vi "mod_QAM Transmitter Gen Symbl Map.vi"(0 "Symbol Rate, Hz":dbl=1.0 format="%.2f", 1 "Reset?":bool=TRUE, 2 "# Samples per Symbol":i32=16, 5 "M-QAM":i32=16, 7 "Message":T3={"# Guard Bits"=4, "# Sync Bits"=40, "# Message Bits"=1000, "PN sequence order"=9}, 9 "System Filter":T2={"TX Filter"=enum."Root Raised Cos", "Alpha"=0.5, "filter length"=8} {"Alpha" format="%.2f"}, 11 "error in (no error)":errorcluster, 12 "Generic Symbol Map Params":T1={"symbol values"=[[1, 17, 21, 5, 4, 20, 16, 0], [33, 49, 53, 37, 36, 52, 48, 32], [41, 57, 61, 45, 44, 60, 56, 40], [9, 25, 29, 13, 12, 28, 24, 8], [11, 27, 31, 15, 14, 30, 26, 10], [43, 59, 63, 47, 46, 62, 58, 42], [35, 51, 55, 39, 38, 54, 50, 34], [3, 19, 23, 7, 6, 22, 18, 2]], "symbol amplitudes (I)"=[-10.0, -8.0, -6.0, -4.0, 4.0, 6.0, 8.0, 10.0], "symbol amplitudes (Q)"=[10.0, 8.0, 6.0, 4.0, -4.0, -6.0, -8.0, -10.0], "gain"=108.0}, 13 "Standard/Generic":enum16{"Standard", "Generic"}(ring)) -> (4 "Output Complex Waveform":T6 {"Y" format="%.3f"; "dt" format="%^.2e"; "t0" format="%.4f"}, 6 "Signal Description":T5 {"QAM System Parameters"."symbol map" format="%.3f"; "matched filter coefficients" format="%.2f"; "pulse shaping filter coefficients" format="%.2f"; "Sync (Symbols)" format="%.2f"}, 15 "error out":errorcluster)   [LabVIEW 2020, in "niDMT.lvlib"]
doc: "This example demonstrates generation of a QAM modulated signal. You can specify characteristics of the message signal such as PN sequence order, number of guard bits, number of sync bits, and transmit filter parameters. You can extend this example to download the generated QAM signal to GPIB-based RF signal generators."
uses:
  <vilib>/addons/Modulation/niDMT.lvlib
  <vilib>/addons/Modulation/Digital/Support/Controls/QAM System Parameters.ctl
  <vilib>/addons/Modulation/Analog/controls/Complex Data Waveform.ctl
  <vilib>/addons/Modulation/Analog/support/mod_Set Error Source.vi
  <vilib>/addons/Modulation/Digital/Support/Common/Validators/mod_Generate Filter Coefficients Validate.vi
  <vilib>/addons/Modulation/Digital/General/subVIs/mod_Generate Filter Coefficients.vi
  <vilib>/addons/Modulation/Digital/General/MT Generate QAM System Parameters(M).vi
  <vilib>/addons/Modulation/niAMT.lvlib
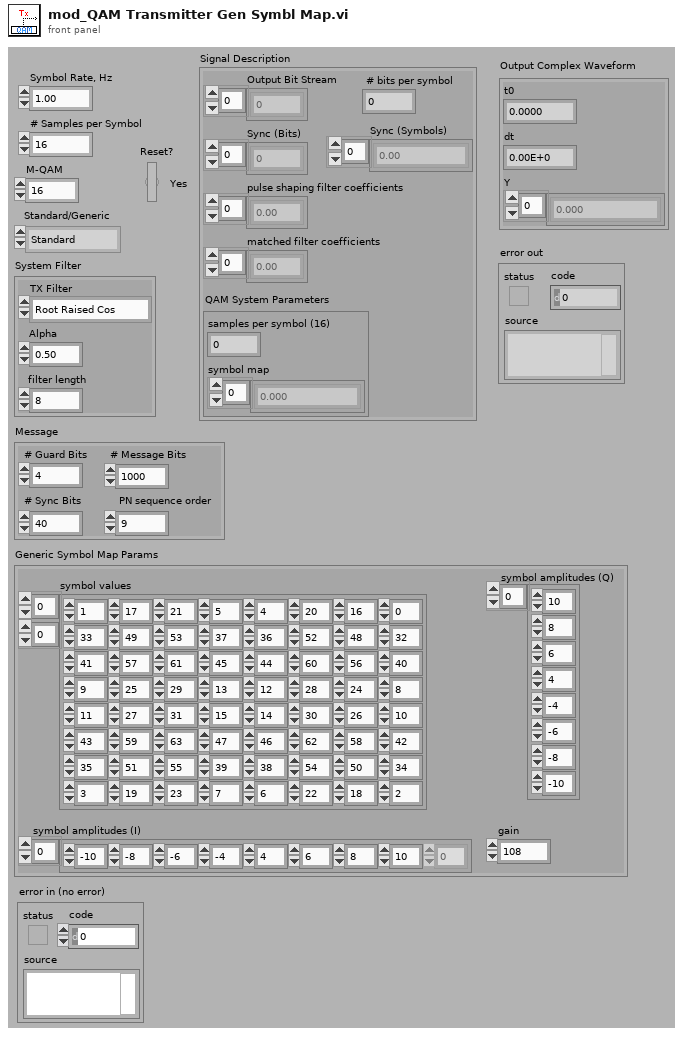
[diagram p1: front panel]
types:
  T1 = cluster{"symbol values":i32[][], "symbol amplitudes (I)":dbl[], "symbol amplitudes (Q)":dbl[], "gain":dbl}
  T2 = cluster{"TX Filter":enum16{"none", "Raised Cosine", "Root Raised Cos", "Gaussian"}, "Alpha":dbl, "filter length":i32}
  T3 = cluster{"# Guard Bits":i32, "# Sync Bits":i32, "# Message Bits":i32, "PN sequence order":i32}
  T4 = typedef "niDMT.lvlib/QAM System Parameters.ctl" = cluster{"samples per symbol (16)":i32, "symbol map":cdb[]}
  T5 = cluster{"Output Bit Stream":i8[], " # bits per symbol":i32, "Sync (Bits)":i8[], "Sync (Symbols)":cdb[], "pulse shaping filter coefficients":dbl[], "matched filter coefficients":dbl[], "QAM System Parameters":T4}
  T6 = typedef "niAMT.lvlib/Complex Data Waveform.ctl" = cluster{"t0":dbl, "dt":dbl, "Y":cdb[]}
  T7 = cluster{"Output Bit Stream":i8[], "# bits per symbol":i32, "Sync (Bits)":i8[], "Sync (Symbols)":cdb[], "pulse shaping filter coefficients":dbl[], "matched filter coefficients":dbl[], "QAM System Parameters":T4}
  T8 = enum16{"none", "Raised Cosine", "Root Raised Cos", "Gaussian"}
  T9 = cluster{"samples per symbol (16)":i32, "symbol map":cdb[]}
  T10 = cluster{"# Samples per Symbol":i32, "symbol map":cdb[]}
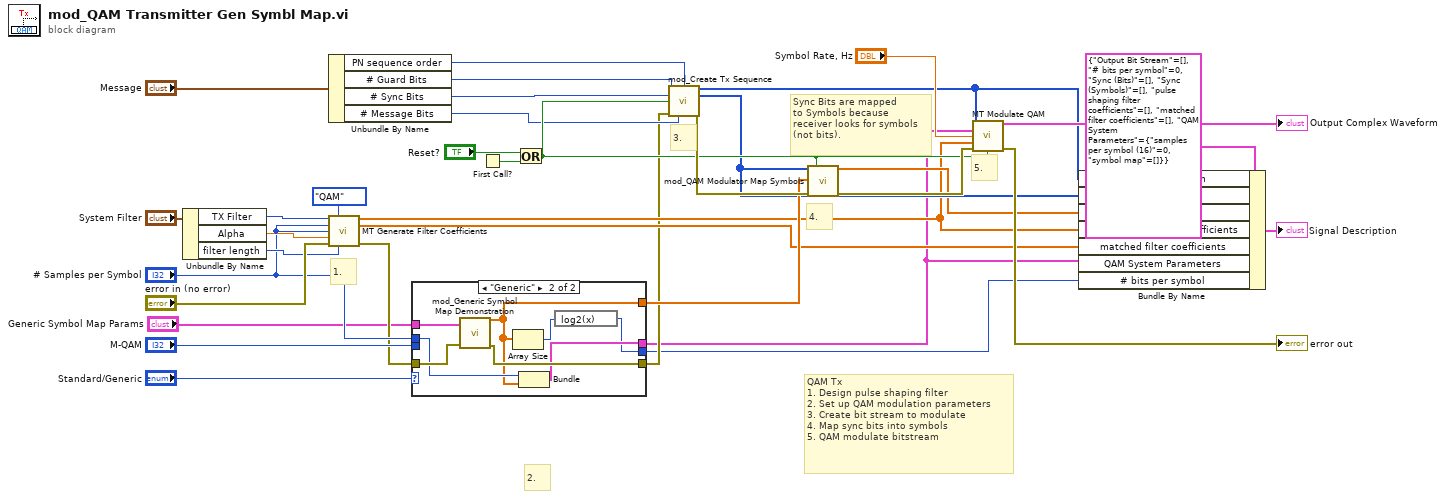
[diagram p0: block diagram]
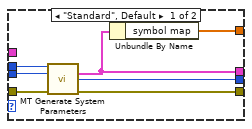
[diagram p2: hidden frame]
diagram:
  # "5."
  # "4."
  # "2."
  # "3."
  # "1."
  # "QAM Tx\n1. Design pulse shaping filter\n2. Set up QAM modulation parameters\n3. Create bit stream to modulate\n4. Map sync bits into symbols\n5. QAM modulate bitstream"
  # "Sync Bits are mapped\nto Symbols because\nreceiver looks for symbols\n(not bits)."
  n1 = Unbundle By Name("System Filter") -> ("TX Filter"=w20:T8, "Alpha"=w19:dbl, "filter length"=w18:i32)
  n2 = Unbundle By Name("Message") -> ("PN sequence order"=w12:i32, "# Guard Bits"=w24:i32, "# Sync Bits"=w23:i32, "# Message Bits"=w22:i32)
  n3 = call <vilib>:"MT Generate Filter Coefficients.vi"("pulse shaping filter (none)"=w20, "modulation type"=enum16{"FSK", "PSK", "QAM", "MSK", "PAM", "ASK"}."QAM", "pulse shaping samples per symbol (16)"="# Samples per Symbol", "matched samples per symbol (16)"="# Samples per Symbol", "filter parameter"=w19, "error in (no error)"="error in (no error)", "filter length (symbols)"=w18) -> ("pulse shaping filter coefficients"=w14:dbl[], "matched filter coefficients"=w13:dbl[], "error out"=w4:errorcluster)  [unwired: 6 out]
  n4 = case shown="\"Generic\"" "Standard/Generic" {
    tunnel: [w42 w44] -> w26
    tunnel: "M-QAM" -> [w41 _]
    tunnel: [w40 w50] -> w8
    tunnel: [w39 w45] -> w7
    tunnel: [w38 w47] -> w2
    tunnel: "# Samples per Symbol" -> [w37 w48]
    tunnel: w4 -> [w36 w49]
    tunnel: "Generic Symbol Map Params" -> [_ w43]
    frame "Standard", Default {
      n5 = call-poly <vilib>:"MT Generate System Parameters.vi"("samples per symbol (16)"=w37, "M-QAM (16)"=w41, "error in (no error)"=w36) -> ("QAM system parameters"=w38:T9, "bits per symbol"=w39:i32, "error out"=w40:errorcluster)  [unwired: 10 out]
      n6 = Unbundle By Name(w38) -> ("symbol map"=w42:cdb[])
    }
    frame "Generic" {
      n7 = call <vilib>:"mod_Generic Symbol Map Demonstration.vi"("Generic Symbol Map Params"=w43, "error in (no error)"=w49) -> ("symbol map"=w44:cdb[], "error out"=w50:errorcluster)  [unwired: 12 out]
      n8 = Array Size(array=w44) -> (size(s)=w46:i32)
      n9 = Bundle("# Samples per Symbol"=w48, "symbol map"=w44) -> (w47:T10)  [unwired: 1 out]
      n10 = expression code="log2(x)"(w46) -> (w45:i32)
    }
  }
  n11 = First Call?() -> (First Call?: T/F=w29:bool)
  n12 = Or(x="Reset?", y=w29) -> (x .or. y?=w27:bool)
  n13 = call <vilib>:"mod_Create Tx Sequence.vi"("# Guard Bits (2)"=w24, "PN sequence order (9)"=w12, "# Sync Bits (20)"=w23, "Reset? (T)"=w27, "error in (no error)"=w8, "# Message Bits"=w22) -> ("Output Bit Stream"=w17:i8[], "Last Sync Pattern"=w16:i8[], "error out"=w33:errorcluster)  [unwired: 3 in, 4 out]
  n14 = call <vilib>:"mod_QAM Modulator Map Symbols.vi"("Input Bit Stream"=w16, "Symbol Map"=w26, "error in (no error)"=w33, "Reset? (T)"=w27) -> ("Symbols"=w15:cdb[], "error out"=w34:errorcluster)  [unwired: 10 out]
  n15 = call <vilib>:"MT Modulate QAM.vi"("input bit stream"=w17, "QAM system parameters"=w2, "symbol rate (Hz)"="Symbol Rate, Hz", "pulse shaping filter coefficients"=w14, "error in (no error)"=w34, "reset? (T)"=w27) -> ("output complex waveform"=→"Output Complex Waveform":T6, "error out"=→"error out":errorcluster)  [unwired: 1 in, 7 out]
  n16 = Bundle By Name(cluster=T7 {"Output Bit Stream"=[], "# bits per symbol"=0, "Sync (Bits)"=[], "Sync (Symbols)"=[], "pulse shaping filter coefficients"=[], "matched filter coefficients"=[], "QAM System Parameters"={"samples per symbol (16)"=0, "symbol map"=[]}} ("Signal Description"), "Output Bit Stream"=w17, "Sync (Bits)"=w16, "Sync (Symbols)"=w15, "pulse shaping filter coefficients"=w14, "matched filter coefficients"=w13, "QAM System Parameters"=w2, "# bits per symbol"=w7) -> (→"Signal Description":T7)
